vi "PWM RGB LED.vi"() -> ()   [LabVIEW 2020, in "CTI-Scratchpad.lvlib"]
uses:
  CTI-Scratchpad.lvlib
  CTI/GPIO Number.ctl
  CTI/Session/Session.lvclass
  CTI/VisaComms/VisaComms.lvclass
  CTI/CTI.lvlib
panel:
  in  "Brightness":sgl(slide) scale=0.0..1.0
  in  "Color":u32(colorbox)
  in  "B GPIO":T1=6
  in  "G GPIO":T1=4
  in  "Port":refnum<visa-resource-name>="COM5"
  in  "R GPIO":T1=2
  in  "stop":bool
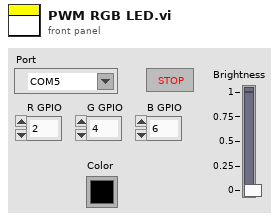
[diagram p1: front panel]
types:
  T1 = typedef "CTI.lvlib/GPIO Number.ctl" = i8
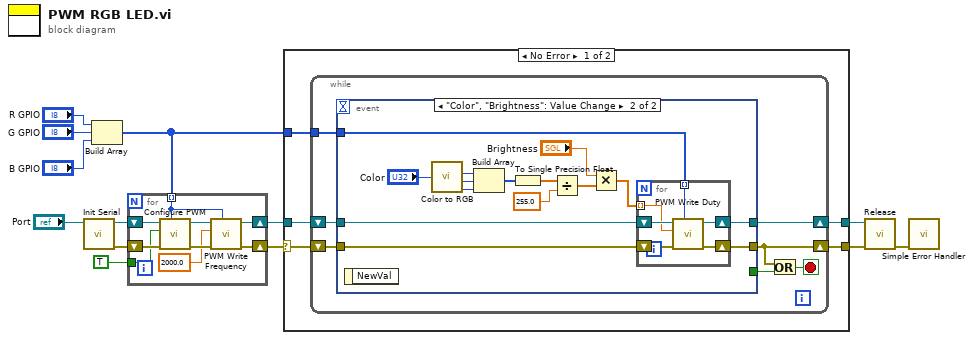
[diagram p0: block diagram]
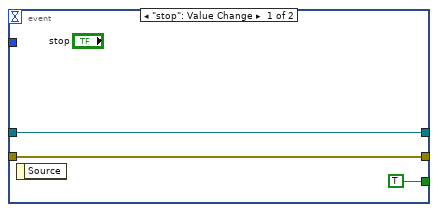
[diagram p2: hidden frame]
diagram:
  n1 = call "Init Serial.vi"("VISA resource name in"="Port") -> ("error out"=w12:errorcluster, "Session"=w13:refnum<class "Session.lvclass">)  [unwired: 8 in, 1 out]
  n2 = Build Array("R GPIO", "G GPIO", "B GPIO") -> (w1:T1[])
  n3 = for {
    tunnel: TRUE ("Enable (F)") -> [w20]
    shift-right: [w15] -> w10
    shift-left: w13 -> [w22]
    shift-right: [w16] -> w11
    shift-left: w12 -> [w21]
    tunnel: w1 -> [w14] mode=indexing
    n4 = call "Configure PWM.vi"("GPIO #"=w14, "error in (no error)"=w21, "Enable (F)"=w20, "Session in"=w22) -> ("error out"=w18:errorcluster, "Session out"=w19:refnum<class "Session.lvclass">)  [unwired: 6 in]
    n5 = call "PWM Write Frequency.vi"("GPIO #"=w14, "error in (no error)"=w18, "Frequency Hz"=sgl 2000.0, "Session in"=w19) -> ("error out"=w16:errorcluster, "Session out"=w15:refnum<class "Session.lvclass">)  [unwired: 6 in]
  }
  n6 = case shown="No Error" w11 {
    selector: w11 -> [w26 w59]
    tunnel: w10 -> [w27 w60]
    tunnel: [w25 w60] -> w8
    tunnel: [w24 w59] -> w9
    tunnel: w1 -> [w23 _]
    frame No Error {
      n7 = while {
        shift-right: [w30] -> w25
        shift-left: w27 -> [w33]
        shift-right: [w29] -> w24
        shift-left: w26 -> [w32]
        tunnel: w23 -> [w28]
        stop <- w34 stop-if-true
        n8 = event shown="[1] \"Color\", \"Brightness\": Value Change" {
          selector: _ -> [_ _]
          dyn-events: _ -> [_ _]
          timeout: _ -> [_ _]
          tunnel: [w37 w50] -> w30
          tunnel: w33 -> [w37 w52]
          tunnel: [w36 w49] -> w29
          tunnel: w32 -> [w36 w51]
          tunnel: [TRUE _] -> w31
          tunnel: w28 -> [_ w41]
          event "stop": Value Change {
            n9 = event-data() -> ()  [unwired: 1 in, 1 out]
          }
          event "Color", "Brightness": Value Change {
            n10 = event-data() -> ()  [unwired: 1 in, 1 out]
            n11 = call <vilib>:"Color to RGB.vi"("Color"="Color") -> ("R"=w48:u8, "G"=w46:u8, "B"=w47:u8)  [unwired: 1 out]
            n12 = Build Array(w48, w46, w47) -> (w45:u8[])
            n13 = To Single Precision Float(number=w45) -> (single precision float=w44:sgl[])
            n14 = Divide(x=w44, y=sgl 255.0) -> (x/y=w42:sgl[])
            n15 = Multiply(x="Brightness", y=w42) -> (x*y=w40:sgl[])
            n16 = for {
              shift-right: [w56] -> w50
              shift-left: w52 -> [w58]
              shift-right: [w55] -> w49
              shift-left: w51 -> [w57]
              tunnel: w40 -> [w54] mode=indexing
              tunnel: w41 -> [w53] mode=indexing
              n17 = call "PWM Write Duty.vi"("GPIO #"=w53, "error in (no error)"=w57, "Duty % (0-1)"=w54, "Session in"=w58) -> ("error out"=w55:errorcluster, "Session out"=w56:refnum<class "Session.lvclass">)  [unwired: 6 in]
            }
          }
        }
        n18 = Or(x=w29, y=w31) -> (x .or. y?=w34:bool)
      }
    }
    frame Error {
    }
  }
  n19 = call-dynamic "Release.vi"("error in (no error)"=w9, "Session in"=w8) -> ("error out"=w7:errorcluster)  [unwired: 9 in]
  n20 = call <vilib>:"Simple Error Handler.vi"("error in (no error)"=w7) -> ()  [unwired: 4 in, 5 out]
